vi "Format Client Request (Notification).vi"(8 "error in (no error)":errorcluster, 9 "id":string, 10 "params":variant, 11 "method":string) -> (0 "error out":errorcluster, 2 "Request String":string)   [LabVIEW 2015, in "JSONRPC Server.lvclass"]
uses:
  JSONRPC Server.lvclass
  <vilib>/NI/i3 JSON/i3-json.lvlib
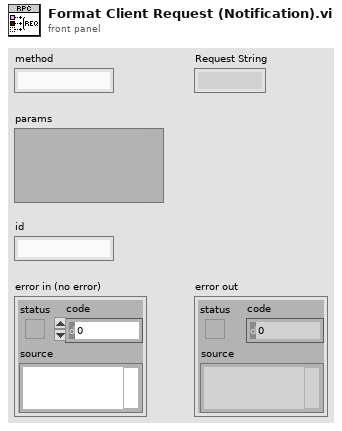
[diagram p1: front panel]
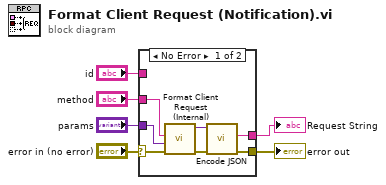
[diagram p0: block diagram]
diagram:
  n1 = case shown="No Error" "error in (no error)" {
    selector: "error in (no error)" -> [w13 w14]
    tunnel: [w12 w14] -> w5
    tunnel: "params" -> [w7 _]
    tunnel: [w11 _] -> w3
    tunnel: "method" -> [w10 _]
    tunnel: "id" -> [_ _]
    frame No Error {
      n2 = call "Format Client Request (Internal).vi"("error in (no error)"=w13, "params"=w7, "method"=w10) -> ("error out"=w8:errorcluster, "JSON Tree out (JSON Object)"=w9:variant)  [unwired: 7 in]
      n3 = call <vilib>:"Encode JSON.vi"("error in (no error)"=w8, "JSON Tree In"=w9) -> ("error out"=w12:errorcluster, "String"=w11:string)  [unwired: 4 in]
    }
    frame Error {
    }
  }
  "error out" <- w5
  "Request String" <- w3
